vi "AddColumn.vi"(8 "error in (no error)":errorcluster, 10 "GridColumn.lvclass":refnum<class "GridColumn.lvclass">, 11 "DataGrid in":refnum<class "DataGridView.lvclass">) -> (0 "error out":errorcluster, 3 "DataGrid out":refnum<class "DataGridView.lvclass">)   [LabVIEW 2014, in "DataGridView.lvclass"]
uses:
  DataGridView.lvclass
  GridColumn/GridColumn.lvclass
  GridColumn/GridColumn.lvclass/GridColumn.ctl
  DataGridView.lvclass/DataGridView.ctl
  System.Windows.Forms
  GridColumn/Read datatype.vi
  GridColumn/Read Name.vi
  GridColumn/Read Params.vi
  GridColumn/Read AutoSizeMode.vi
  GridColumn/Read FillWeight.vi
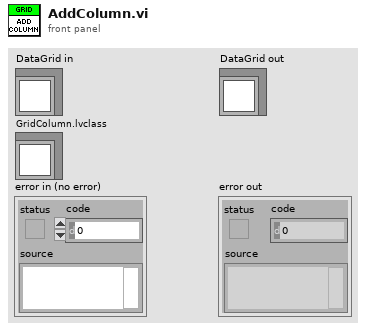
[diagram p1: front panel]
types:
  T1 = enum16{"string", "image", "link", "check", "combo", "button"}
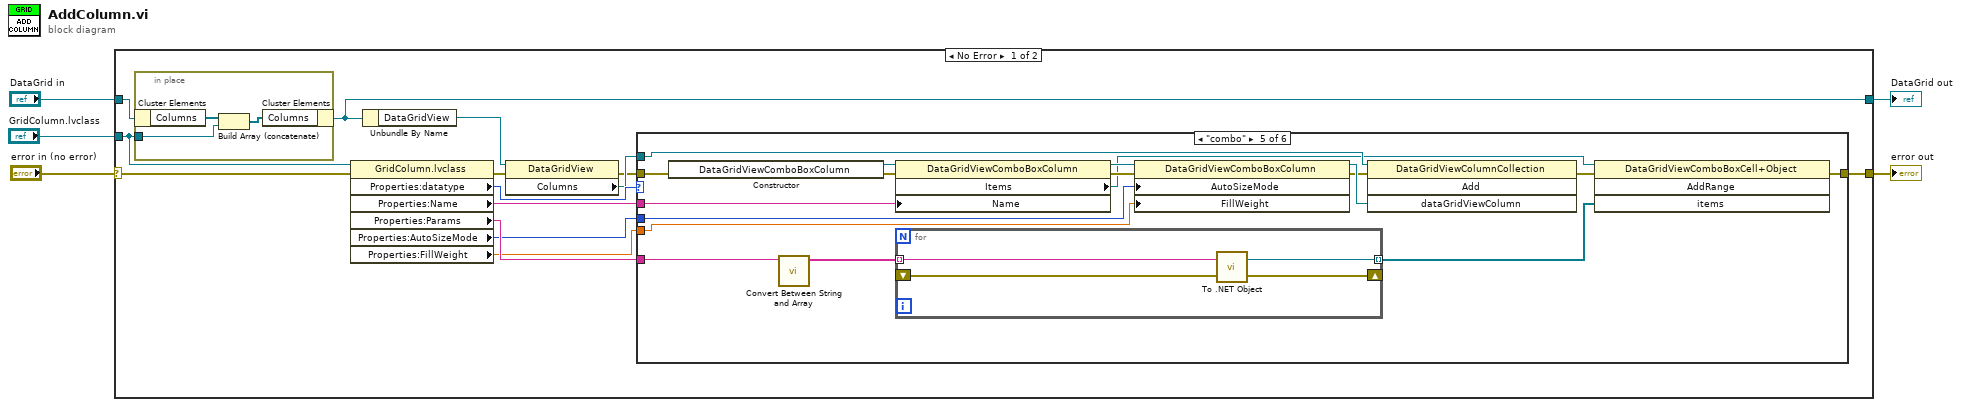
[diagram p0: block diagram]
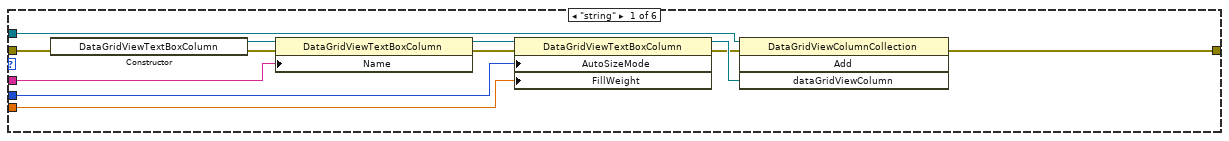
[diagram p2: hidden frame]
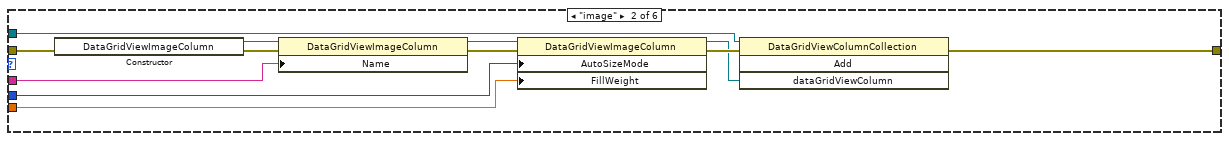
[diagram p3: hidden frame]
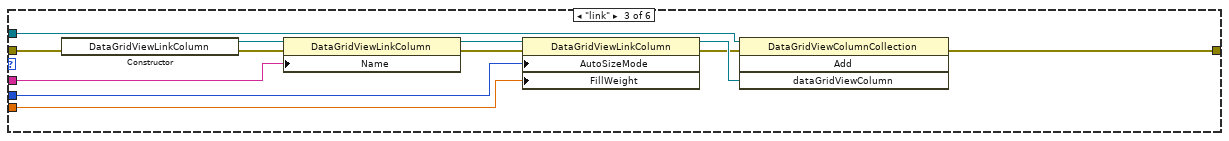
[diagram p4: hidden frame]
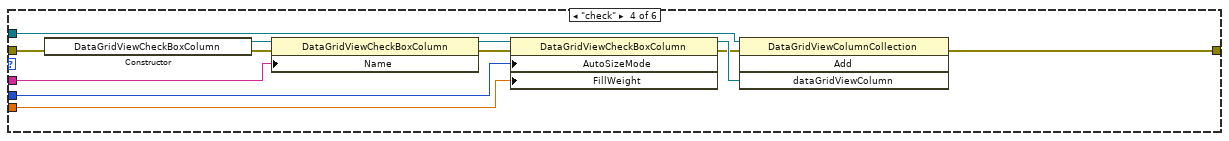
[diagram p5: hidden frame]
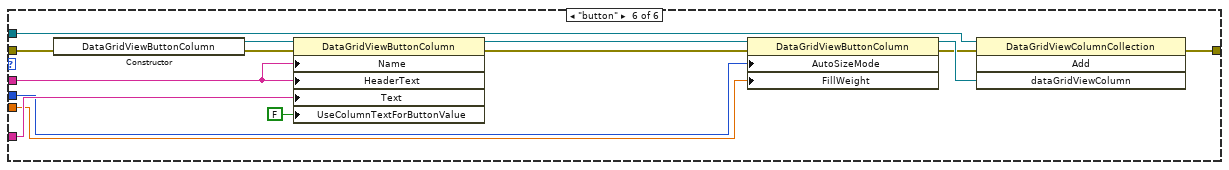
[diagram p6: hidden frame]
diagram:
  n1 = case shown="No Error" "error in (no error)" {
    selector: "error in (no error)" -> [w13 w107]
    tunnel: [w10 w107] -> w4
    tunnel: [w17 w106] -> w2
    tunnel: "DataGrid in" -> [w19 w106]
    tunnel: "GridColumn.lvclass" -> [w18 _]
    frame No Error {
      n2 = in-place {
        in-place-border: w18 -> [w104]
        n3 = in-place-cluster #1(w19) -> ("Columns"=w105:refnum<class "GridColumn.lvclass">[])
        n4 = Build Array (concatenate)(w105, w104) -> (w103:refnum<class "GridColumn.lvclass">[])
        n5 = in-place-cluster #1("Columns"=w103) -> (w17:refnum<class "DataGridView.lvclass">)
      }
      n6 = property class="GridColumn.lvclass"(reference=w18, error in=w13) -> (error out=w12:errorcluster, "Properties:datatype"=w16:T1, "Properties:Name"=w14:string, "Properties:Params"=w9:string, "Properties:AutoSizeMode"=w8:i32, "Properties:FillWeight"=w7:sgl)  [unwired: 1 out]
      n7 = Unbundle By Name(w17) -> ("DataGridView"=w6:refnum<k24>)
      n8 = property class="DataGridView"(reference=w6, error in=w12) -> (error out=w11:errorcluster, "Columns"=w15:refnum<k24>)  [unwired: 1 out]
      n9 = case shown="\"combo\"" w16 {
        tunnel: w15 -> [w31 w43 w55 w67 w84 w102]
        tunnel: w14 -> [w29 w40 w52 w64 w77 w97]
        tunnel: w11 -> [w26 w39 w51 w63 w81 w99]
        tunnel: [w27 w38 w50 w62 w75 w98] -> w10
        tunnel: w9 -> [_ _ _ _ w78 w96]
        tunnel: w8 -> [w21 w33 w48 w57 w69 w94]
        tunnel: w7 -> [w20 w32 w47 w56 w68 w93]
        frame "string" {
          n10 = constructor class="DataGridViewTextBoxColumn"(error in=w26) -> (reference out=w30:refnum<k24>, error out=w28:errorcluster)  [unwired: 2 in, 1 out]
          n11 = property class="DataGridViewTextBoxColumn"(reference=w30, error in=w28, "Name"=w29) -> (reference out=w25:refnum<k24>, error out=w24:errorcluster)
          n12 = property class="DataGridViewTextBoxColumn"(reference=w25, error in=w24, "AutoSizeMode"=w21, "FillWeight"=w20) -> (reference out=w23:refnum<k24>, error out=w22:errorcluster)
          n13 = invoke class="DataGridViewColumnCollection" method="Add"(reference=w31, error in=w22, "dataGridViewColumn"=w23) -> (error out=w27:errorcluster)  [unwired: 1 in, 3 out]
        }
        frame "image" {
          n14 = constructor class="DataGridViewImageColumn"(error in=w39) -> (reference out=w42:refnum<k24>, error out=w41:errorcluster)  [unwired: 2 in, 1 out]
          n15 = property class="DataGridViewImageColumn"(reference=w42, error in=w41, "Name"=w40) -> (reference out=w37:refnum<k24>, error out=w36:errorcluster)
          n16 = property class="DataGridViewImageColumn"(reference=w37, error in=w36, "AutoSizeMode"=w33, "FillWeight"=w32) -> (reference out=w34:refnum<k24>, error out=w35:errorcluster)
          n17 = invoke class="DataGridViewColumnCollection" method="Add"(reference=w43, error in=w35, "dataGridViewColumn"=w34) -> (error out=w38:errorcluster)  [unwired: 1 in, 3 out]
        }
        frame "link" {
          n18 = constructor class="DataGridViewLinkColumn"(error in=w51) -> (reference out=w54:refnum<k24>, error out=w53:errorcluster)  [unwired: 2 in, 1 out]
          n19 = property class="DataGridViewLinkColumn"(reference=w54, error in=w53, "Name"=w52) -> (reference out=w46:refnum<k24>, error out=w49:errorcluster)
          n20 = property class="DataGridViewLinkColumn"(reference=w46, error in=w49, "AutoSizeMode"=w48, "FillWeight"=w47) -> (reference out=w45:refnum<k24>, error out=w44:errorcluster)
          n21 = invoke class="DataGridViewColumnCollection" method="Add"(reference=w55, error in=w44, "dataGridViewColumn"=w45) -> (error out=w50:errorcluster)  [unwired: 1 in, 3 out]
        }
        frame "check" {
          n22 = constructor class="DataGridViewCheckBoxColumn"(error in=w63) -> (reference out=w66:refnum<k24>, error out=w65:errorcluster)  [unwired: 2 in, 1 out]
          n23 = property class="DataGridViewCheckBoxColumn"(reference=w66, error in=w65, "Name"=w64) -> (reference out=w61:refnum<k24>, error out=w60:errorcluster)
          n24 = property class="DataGridViewCheckBoxColumn"(reference=w61, error in=w60, "AutoSizeMode"=w57, "FillWeight"=w56) -> (reference out=w59:refnum<k24>, error out=w58:errorcluster)
          n25 = invoke class="DataGridViewColumnCollection" method="Add"(reference=w67, error in=w58, "dataGridViewColumn"=w59) -> (error out=w62:errorcluster)  [unwired: 1 in, 3 out]
        }
        frame "combo" {
          n26 = constructor class="DataGridViewComboBoxColumn"(error in=w81) -> (reference out=w83:refnum<k24>, error out=w82:errorcluster)  [unwired: 2 in, 1 out]
          n27 = call "Convert Between String and Array.vi"("String"=w78) -> ("String Array"=w80:string[])  [unwired: 9 in, 1 out]
          n28 = property class="DataGridViewComboBoxColumn"(reference=w83, error in=w82, "Name"=w77) -> (reference out=w74:refnum<k24>, error out=w73:errorcluster, "Items"=w71:refnum<k24>)
          n29 = for {
            tunnel: [w88] -> w79 mode=indexing
            tunnel: w80 -> [w87] mode=indexing
            shift-right: [w86] -> _
            shift-left: _ -> [w85]
            n30 = call <vilib>:"To .NET Object.vi"("error in (no error)"=w85, "anything"=w87) -> ("error out"=w86:errorcluster, ".NET object"=w88:refnum<k24>)
          }
          n31 = property class="DataGridViewComboBoxColumn"(reference=w74, error in=w73, "AutoSizeMode"=w69, "FillWeight"=w68) -> (reference out=w72:refnum<k24>, error out=w70:errorcluster)
          n32 = invoke class="DataGridViewColumnCollection" method="Add"(reference=w84, error in=w70, "dataGridViewColumn"=w72) -> (error out=w76:errorcluster)  [unwired: 1 in, 3 out]
          n33 = invoke class="DataGridViewComboBoxCell+Object" method="AddRange"(reference=w71, error in=w76, "items"=w79) -> (error out=w75:errorcluster)  [unwired: 1 in, 3 out]
        }
        frame "button" {
          n34 = constructor class="DataGridViewButtonColumn"(error in=w99) -> (reference out=w101:refnum<k24>, error out=w100:errorcluster)  [unwired: 2 in, 1 out]
          n35 = property class="DataGridViewButtonColumn"(reference=w101, error in=w100, "Name"=w97, "HeaderText"=w97, "Text"=w96, "UseColumnTextForButtonValue"=FALSE) -> (reference out=w92:refnum<k24>, error out=w91:errorcluster)
          n36 = property class="DataGridViewButtonColumn"(reference=w92, error in=w91, "AutoSizeMode"=w94, "FillWeight"=w93) -> (reference out=w90:refnum<k24>, error out=w89:errorcluster)
          n37 = invoke class="DataGridViewColumnCollection" method="Add"(reference=w102, error in=w89, "dataGridViewColumn"=w90) -> (error out=w98:errorcluster)  [unwired: 1 in, 3 out]
        }
      }
    }
    frame Error {
    }
  }
  "error out" <- w4
  "DataGrid out" <- w2
